vi "Get Environment Readings from Viewer.vi"(0 "Data URL":string="http://127.0.0.1:12346/latest") -> (2 "String output":string)   [LabVIEW 2020]
uses:
  <vilib>/httpClient/LabVIEWHTTPClient.lvlib
  <vilib>/xml/NI_XML.lvlib
  <resource>/objmgr/DOMUserDefRef.rc
panel:
  out "Parse Errors":string
  out "XML error out":errorcluster
  out "Response body":string
  out "HTTP error out":errorcluster
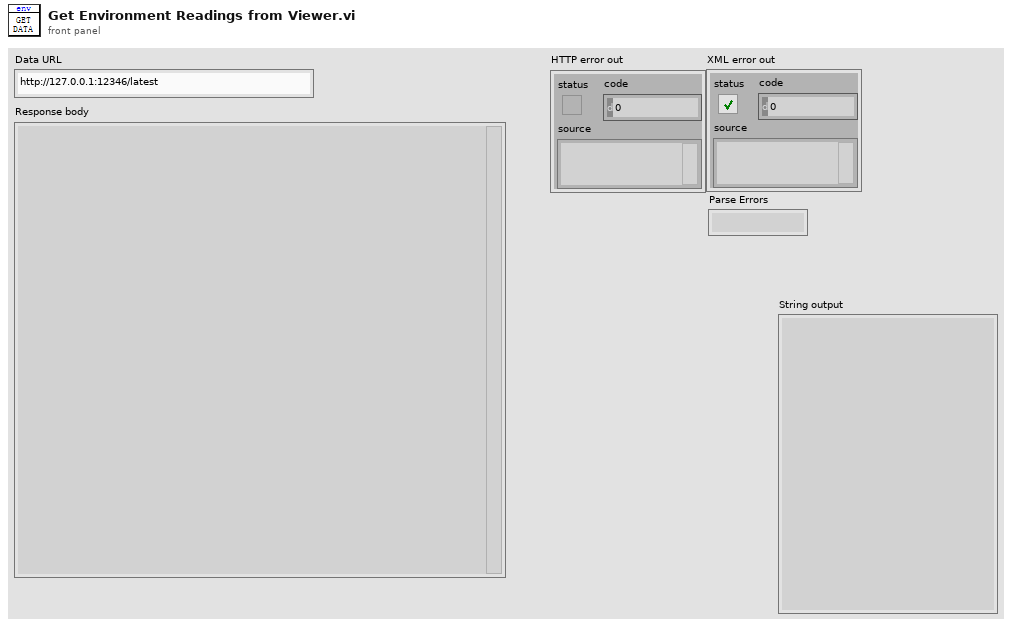
[diagram p1: front panel]
types:
  T1 = cluster{"time":string, "temperature":dbl, "device":string, "humidity":dbl, "altitude":dbl, "pressure":dbl}
  T2 = typedef "LabVIEWHTTPClient.lvlib/ClientHandle.ctl" = refnum<k1>
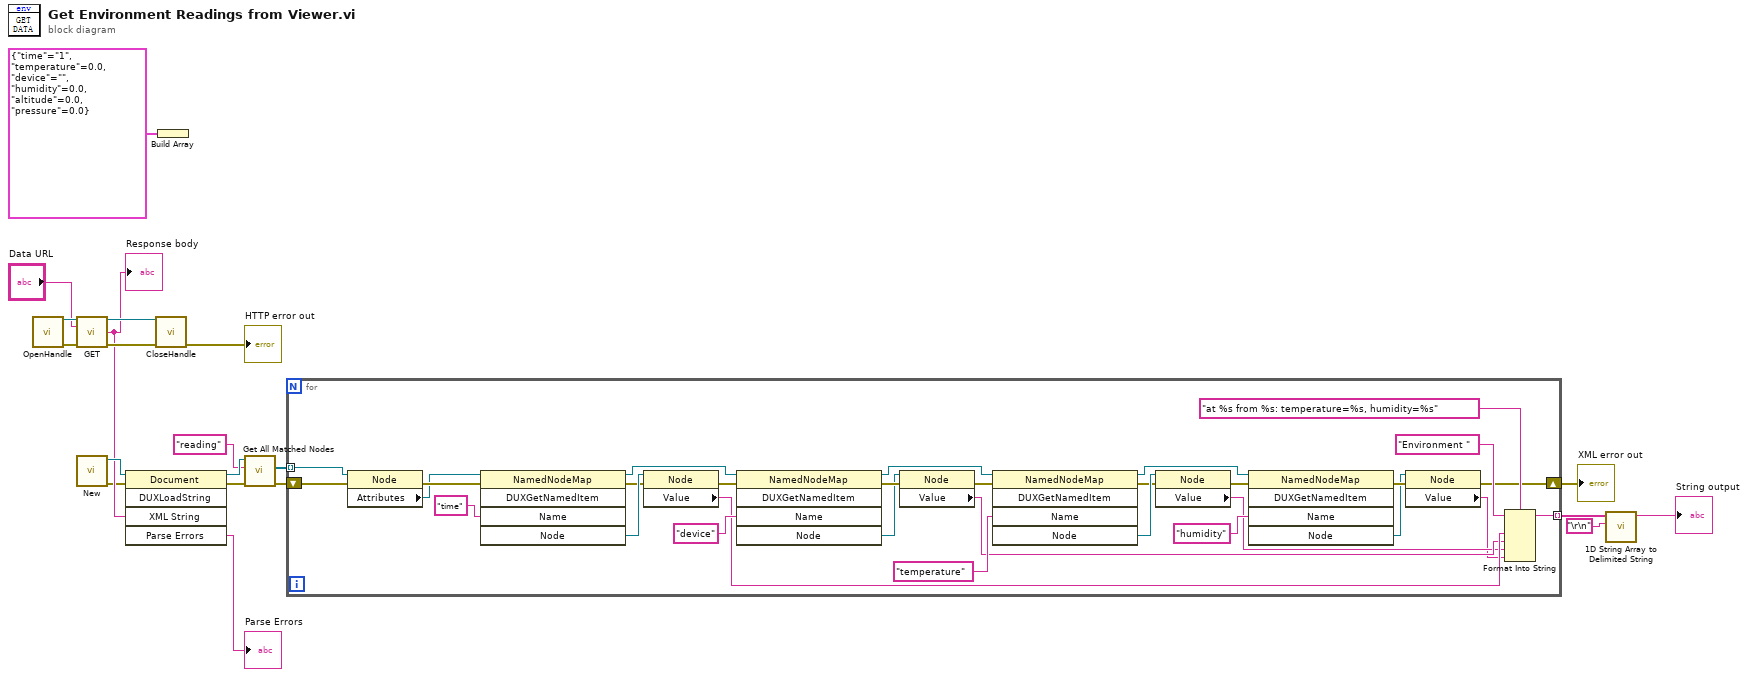
[diagram p0: block diagram]
diagram:
  n1 = call <vilib>:"OpenHandle.vi"() -> ("client handle out"=w20:T2, "error out"=w17:errorcluster)  [unwired: 14 in]
  n2 = call <vilib>:"GET.vi"("client handle"=w20, "url"="Data URL", "error in (no error)"=w17) -> ("client handle out"=w19:T2, "body"=w9:string, "error out"=w18:errorcluster)  [unwired: 9 in, 1 out]
  "Response body" <- w9
  n3 = call <vilib>:"New.vi"() -> ("error out"=w8:errorcluster, "DOM document out"=w10:refnum<k20>)  [unwired: 8 in]
  n4 = invoke class="Document" method="DUXLoadString"(reference=w10, error in=w8, "XML String"=w9) -> (reference out=w6:refnum<k20>, error out=w5:errorcluster, "Parse Errors"=→"Parse Errors":string)  [unwired: 2 in, 2 out]
  n5 = call <vilib>:"CloseHandle.vi"("client handle"=w19, "error in (no error)"=w18) -> ("error out"=→"HTTP error out":errorcluster)  [unwired: 13 in]
  n6 = Build Array(T1 {"time"="1", "temperature"=0.0, "device"="", "humidity"=0.0, "altitude"=0.0, "pressure"=0.0}) -> ()  [unwired: 1 out]
  n7 = call <vilib>:"Get All Matched Nodes.vi"("error in (no error)"=w5, "XPath expression"="reading", "node in"=w6) -> ("error out"=w2:errorcluster, "node result array"=w3:refnum<k20>[])  [unwired: 6 in, 1 out]
  n8 = for {
    tunnel: w3 -> [w47] mode=indexing
    tunnel: [w48] -> w13 mode=indexing
    shift-right: [w32] -> w1
    shift-left: w2 -> [w46]
    n9 = property class="Node"(reference=w47, error in=w46) -> (error out=w43:errorcluster, "Attributes"=w21:refnum<k20>)  [unwired: 1 out]
    n10 = invoke class="NamedNodeMap" method="DUXGetNamedItem"(reference=w21, error in=w43, "Name"="time" ("Get Named Item")) -> (reference out=w24:refnum<k20>, error out=w42:errorcluster, "Node"=w44:refnum<k20>)  [unwired: 2 in, 2 out]
    n11 = property class="Node"(reference=w44, error in=w42) -> (error out=w35:errorcluster, "Value"=w28:string)  [unwired: 1 out]
    n12 = invoke class="NamedNodeMap" method="DUXGetNamedItem"(reference=w24, error in=w35, "Name"="device" ("Get Named Item")) -> (reference out=w23:refnum<k20>, error out=w41:errorcluster, "Node"=w40:refnum<k20>)  [unwired: 2 in, 2 out]
    n13 = property class="Node"(reference=w40, error in=w41) -> (error out=w34:errorcluster, "Value"=w27:string)  [unwired: 1 out]
    n14 = invoke class="NamedNodeMap" method="DUXGetNamedItem"(reference=w23, error in=w34, "Name"="temperature" ("Get Named Item")) -> (reference out=w22:refnum<k20>, error out=w38:errorcluster, "Node"=w39:refnum<k20>)  [unwired: 2 in, 2 out]
    n15 = property class="Node"(reference=w39, error in=w38) -> (error out=w33:errorcluster, "Value"=w26:string)  [unwired: 1 out]
    n16 = invoke class="NamedNodeMap" method="DUXGetNamedItem"(reference=w22, error in=w33, "Name"="humidity" ("Get Named Item")) -> (error out=w37:errorcluster, "Node"=w36:refnum<k20>)  [unwired: 2 in, 3 out]
    n17 = property class="Node"(reference=w36, error in=w37) -> (error out=w32:errorcluster, "Value"=w25:string)  [unwired: 1 out]
    n18 = Format Into String(format string="at %s from %s: temperature=%s, humidity=%s", initial string="Environment ", w28, w27, w26, w25) -> (resulting string=w48:string)  [unwired: 1 in, 1 out]
  }
  "XML error out" <- w1
  n19 = call <vilib>:"1D String Array to Delimited String.vi"("delimiter"="\r\n", "string array"=w13) -> ("delimited string"=→"String output":string)  [unwired: 9 in]
